vi "TestLabjackStream.vi"() -> ()   [LabVIEW 2013]
panel:
  out "?":i32(graph)
  out "?":dbl(graph)
  in  "Delta":dbl=0.1
  out "Number of Triggers":i32
  in  "?":bool
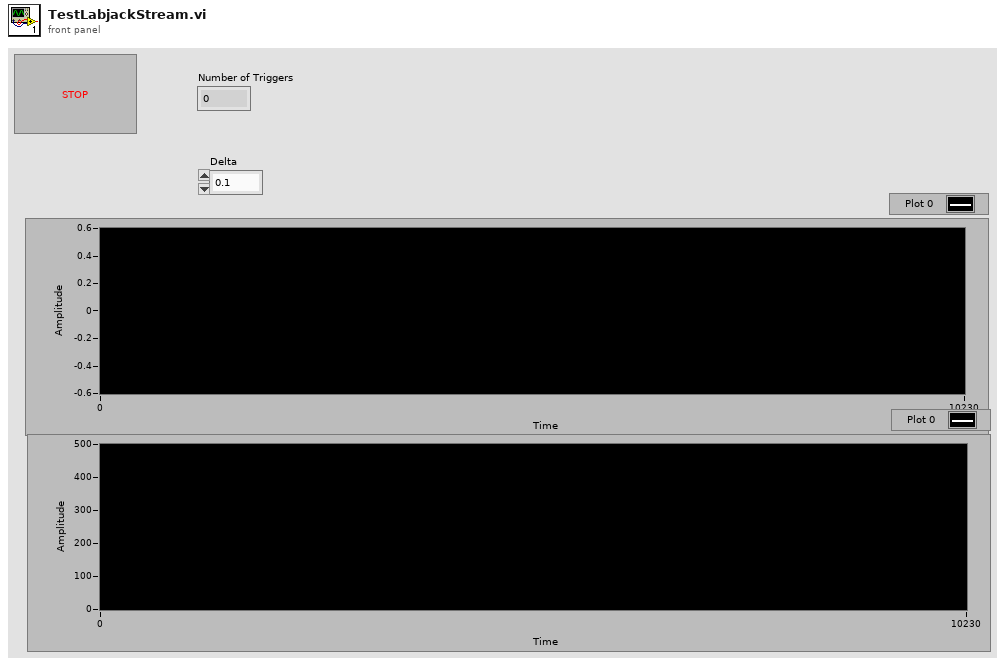
[diagram p1: front panel]
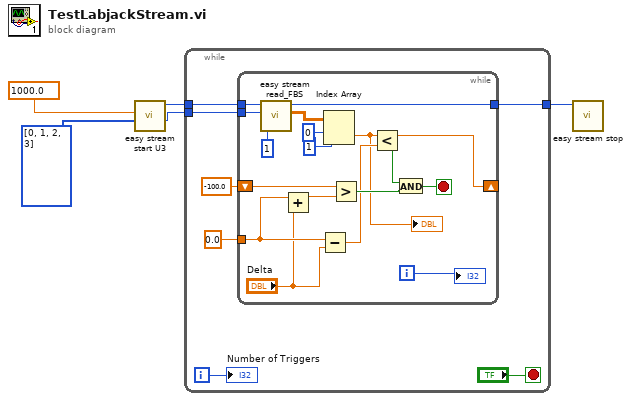
[diagram p0: block diagram]
diagram:
  n1 = call "easy stream start U3.vi"("Scan List (+)"=u8[] [0, 1, 2, 3], "Scan Rate (Hz)"=1000.0) -> ("# Channels"=w1:i32, "Handle Out"=w2:i32)  [unwired: 6 in, 2 out]
  n2 = while {
    tunnel: [w11] -> w5
    tunnel: w2 -> [w10]
    tunnel: w1 -> [w9]
    i -> [w6]
    stop <- "?" stop-if-true
    n3 = while {
      tunnel: [w25] -> w11
      tunnel: w10 -> [w24]
      tunnel: w9 -> [w23]
      shift-right: [w15] -> _
      shift-left: -100.0 -> [w22]
      tunnel: 0.0 -> [w18]
      i -> [w13]
      stop <- w14 stop-if-true
      n4 = call "easy stream read_FBS.vi"("Scans To Read"=1, "# Channels In Stream"=w23, "Handle In"=w24) -> ("Data"=w27:dbl[][], "Handle Out"=w25:i32)  [unwired: 5 in, 2 out]
      n5 = Add(x=w18, y="Delta") -> (x+y=w19:dbl)
      n6 = Subtract(x=w18, y="Delta") -> (x-y=w16:dbl)
      n7 = Index Array(array=w27, index (row)=0, index (col)=1 ("disabled index (col)")) -> (element=w15:dbl)
      "?" <- w15
      n8 = Greater?(x=w22, y=w19) -> (0:w21:bool)
      n9 = Less?(x=w15, y=w16) -> (x < y?=w20:bool)
      n10 = And(x=w20, y=w21) -> (x .and. y?=w14:bool)
      "?" <- w13
    }
    "Number of Triggers" <- w6
  }
  n11 = call "easy stream stop.vi"("Handle In"=w5) -> ()  [unwired: 8 in, 3 out]
